vi "valuation.vi"(0 "Input pixmap":i32[][](array[numeric]), 1 "Ref. N.":i32) -> (2 "4-bit pixmap 3":u8[][](array[numeric])=[[0, 0, 0, 0, 0, 0, 0, 0, 0, 0, 0, 0, 0, 0, 0, 0, 0, 0, 0, 0, 0, 0, 0], [0, 0, 0, 0, 0, 1, 1, 1, 1, 1, 0, 0, 0, 0, 0, 0, 1, 1, 1, 1, 1, 1, 0], [0, 0, 0, 0, 1, 1, 1, 1, 1, 1, 1, 1, 0, 0, 0, 1, 1, 1, 1, 1, 1, 1, 0], [0, 0, 0, 1, 1, 1, 1, 1, 1, 1, 1, 1, 1, 0, 1, 1, 1, 1, 1, 1, 1, 1, 0], [0, 0, 1, 1, 1, 1, 0, 0, 0, 1, 1, 1, 1, 0, 1, 1, 1, 1, 0, 0, 0, 0, 0], [0, 0, 1, 1, 1, 1, 0, 0, 0, 1, 1, 1, 1, 0, 1, 1, 1, 0, 0, 0, 0, 0, 0], [0, 0, 1, 1, 1, 1, 0, 0, 0, 1, 1, 1, 1, 1, 1, 1, 1, 1, 1, 1, 0, 0, 0], [0, 0, 1, 1, 1, 1, 0, 0, 0, 1, 1, 1, 1, 1, 1, 1, 1, 1, 1, 1, 1, 0, 0], [0, 0, 1, 1, 1, 1, 1, 1, 1, 1, 1, 1, 0, 1, 1, 0, 0, 1, 1, 1, 1, 1, 0], [0, 0, 0, 1, 1, 1, 1, 1, 1, 1, 1, 1, 0, 0, 0, 0, 0, 0, 1, 1, 1, 1, 0], [0, 0, 0, 0, 0, 1, 1, 1, 1, 1, 1, 0, 0, 0, 0, 0, 0, 0, 1, 1, 1, 1, 0], [0, 0, 0, 0, 0, 0, 1, 1, 1, 1, 0, 0, 1, 0, 0, 0, 0, 0, 1, 1, 1, 1, 0], [0, 0, 0, 0, 0, 1, 1, 1, 1, 0, 0, 1, 1, 1, 1, 0, 0, 1, 1, 1, 1, 0, 0], [0, 0, 0, 0, 1, 1, 1, 1, 0, 0, 0, 1, 1, 1, 1, 1, 1, 1, 1, 1, 1, 0, 0], [0, 0, 0, 0, 1, 1, 1, 0, 0, 0, 0, 0, 1, 1, 1, 1, 1, 1, 1, 1, 0, 0, 0], [0, 0, 0, 0, 0, 0, 0, 0, 0, 0, 0, 0, 0, 0, 0, 0, 0, 0, 0, 0, 0, 0, 0], [0, 0, 0, 0, 0, 0, 0, 0, 0, 0, 0, 0, 0, 0, 0, 0, 0, 0, 0, 0, 0, 0, 0], [0, 0, 0, 0, 0, 0, 0, 0, 0, 0, 0, 0, 0, 0, 0, 0, 0, 0, 0, 0, 0, 0, 0], [0, 0, 0, 0, 0, 0, 0, 0, 0, 0, 0, 0, 0, 0, 0, 0, 0, 0, 0, 0, 0, 0, 0]] caption="ref. Number" format="%#.1f", 4 "ref. picture":picture caption="ref. pic.", 5 "matched pixmap":i32[][](array[numeric]), 6 "total identify %":dbl format="%#_3g", 7 "vertical × yoko":i32[](array[numeric]))   [LabVIEW 2016]
uses:
  <vilib>/picture/picture.llb/imagedata.ctl
panel:
  out "image data 2":T1 caption="画像データ"
  in  "value method":bool
  in  "タブ制御器":enum32{"picture", "array", "expand"}(tab)
  out "input picture 2":picture caption="Input pic."
  out "new picture":picture caption="matched pic."
  out "image data":T1 caption="画像データ"
  out "input data":T1 caption="画像データ"
  out "map N":i32
  out "sample blackN":i32
  out "ref. data 2":T1 caption="画像データ"
  out "Ref. blackN":i32
  out "sample     ref.  identify":dbl[](array[numeric]) format="%#_3g"
  out "new picture 2":picture caption="falsepix pic."
  out "Expand test pic. 3":picture caption="naname Expanded pic."
  out "unmatched pixmap":i32[][](array[numeric])
  # "1/0"
  # "updown"
  # "="
  # "white : matched\nyellow : only samp. \nblack : only Ref."
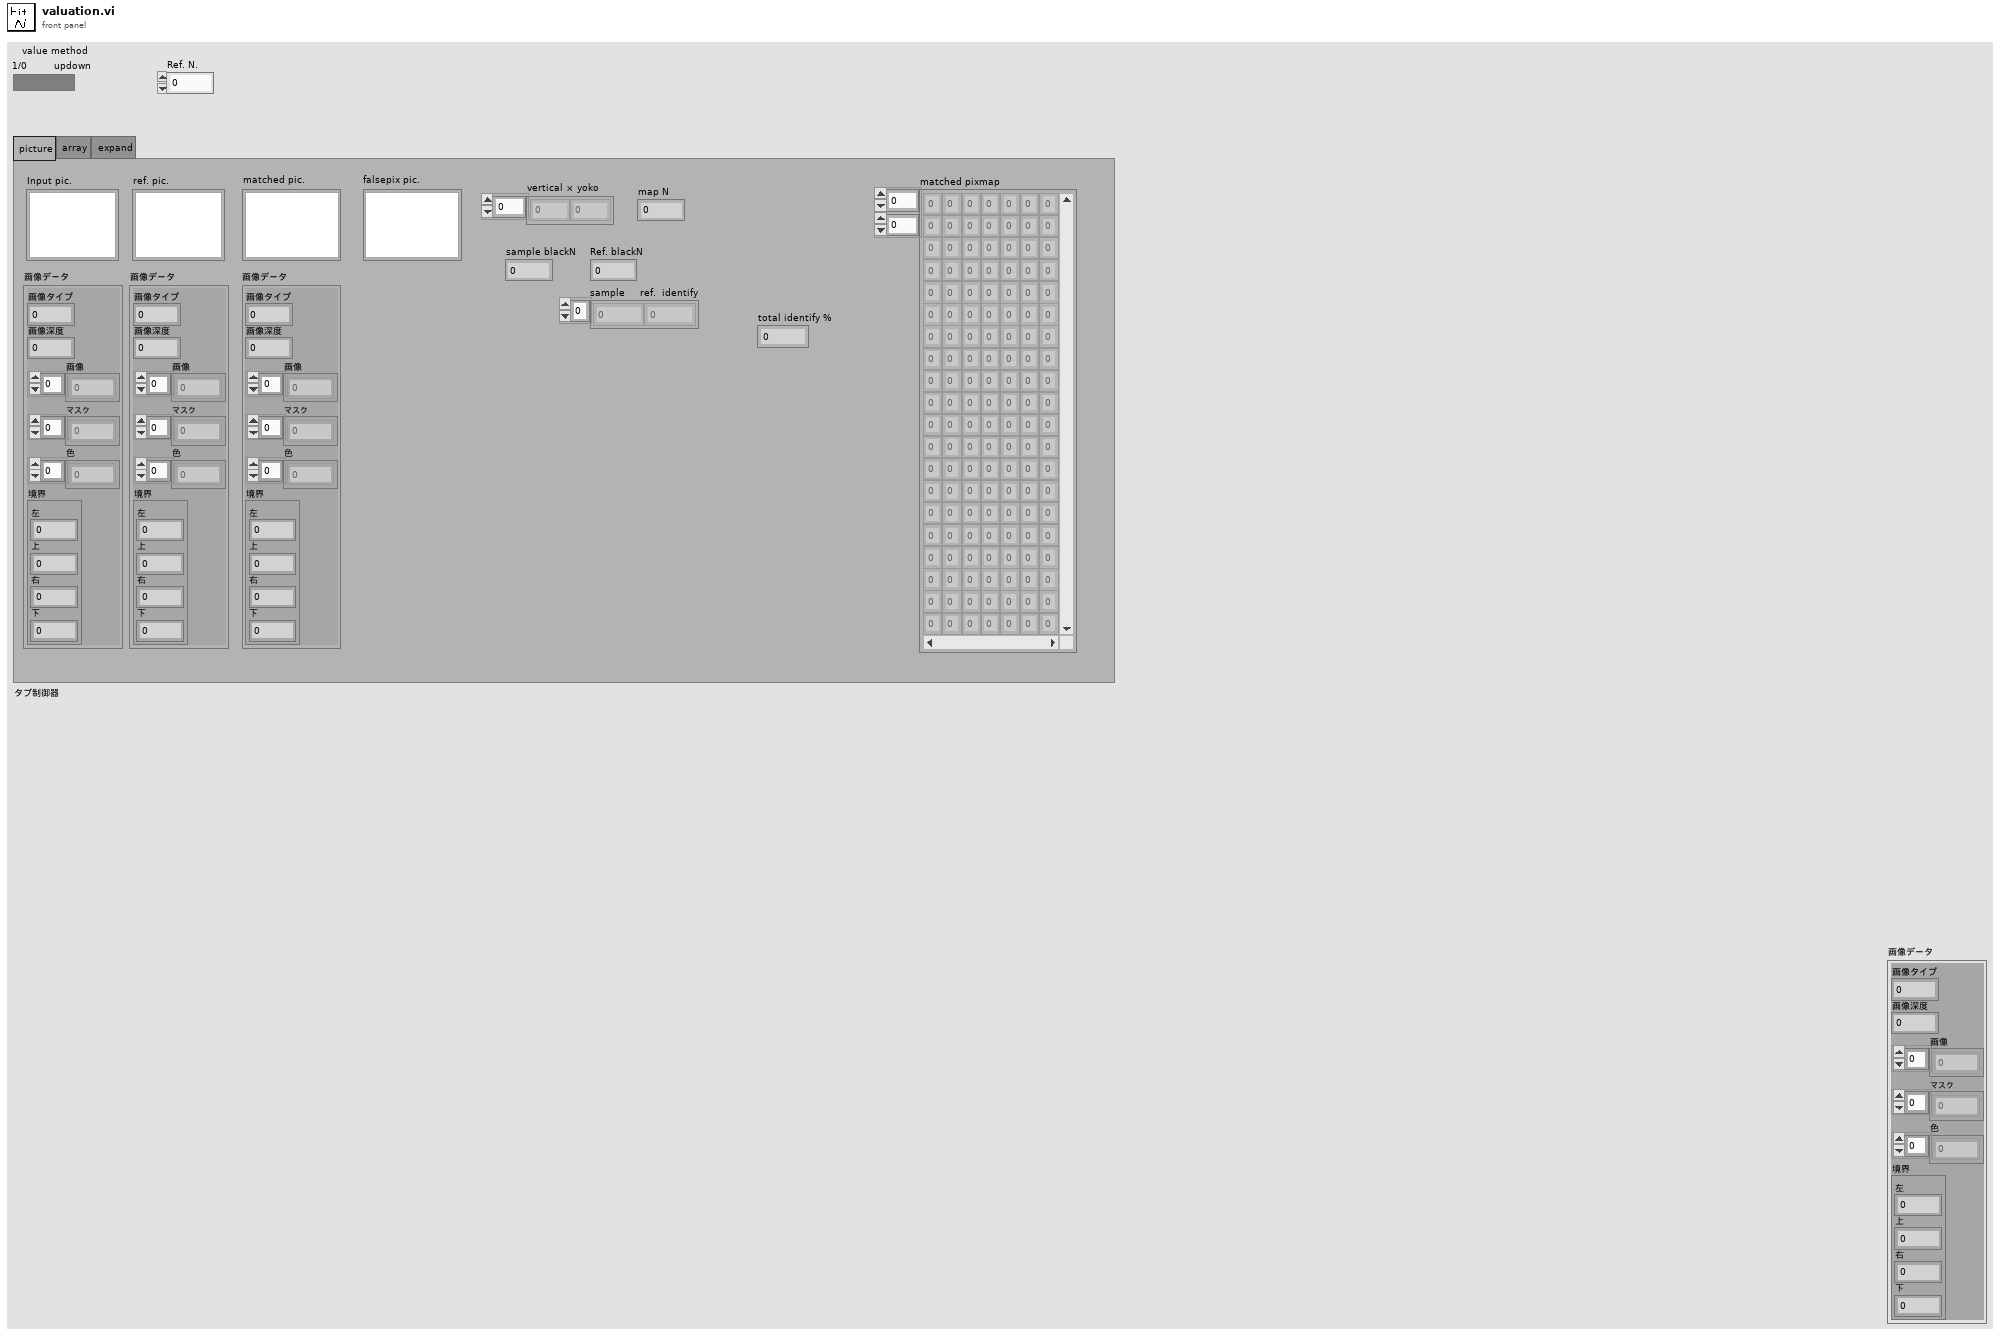
[diagram p1: front panel]
types:
  T1 = typedef "imagedata.ctl" = cluster{"image type":i32, "image depth":i32, "image":u8[], "mask":u8[], "colors":u32[], "Rectangle":cluster{"left":i16, "top":i16, "right":i16, "bottom":i16}}
  T2 = typedef "LVBoundsTypeDef.ctl" = cluster{"Width":u32, "Height":u32}
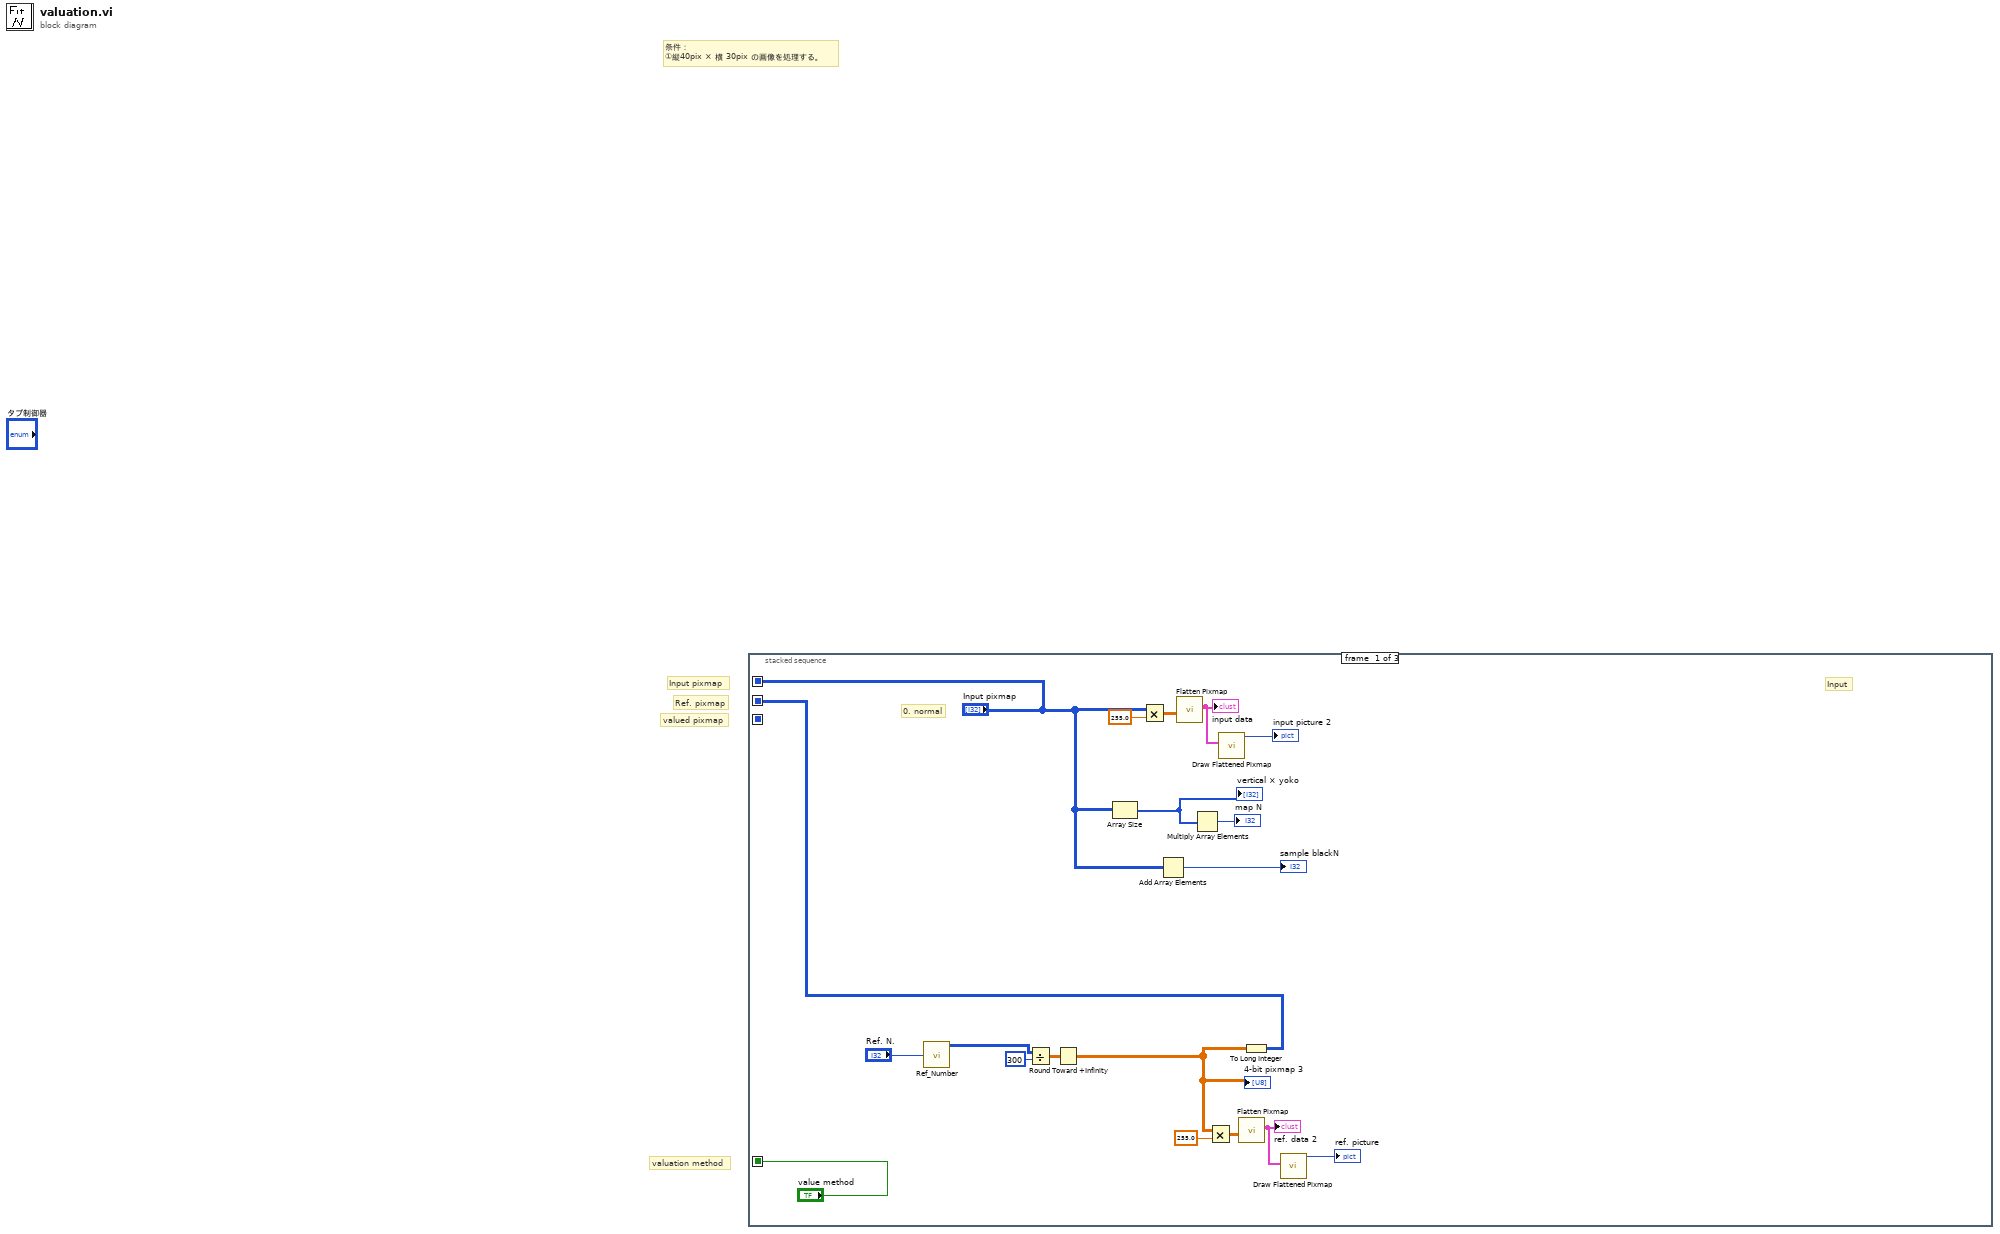
[diagram p0: block diagram]
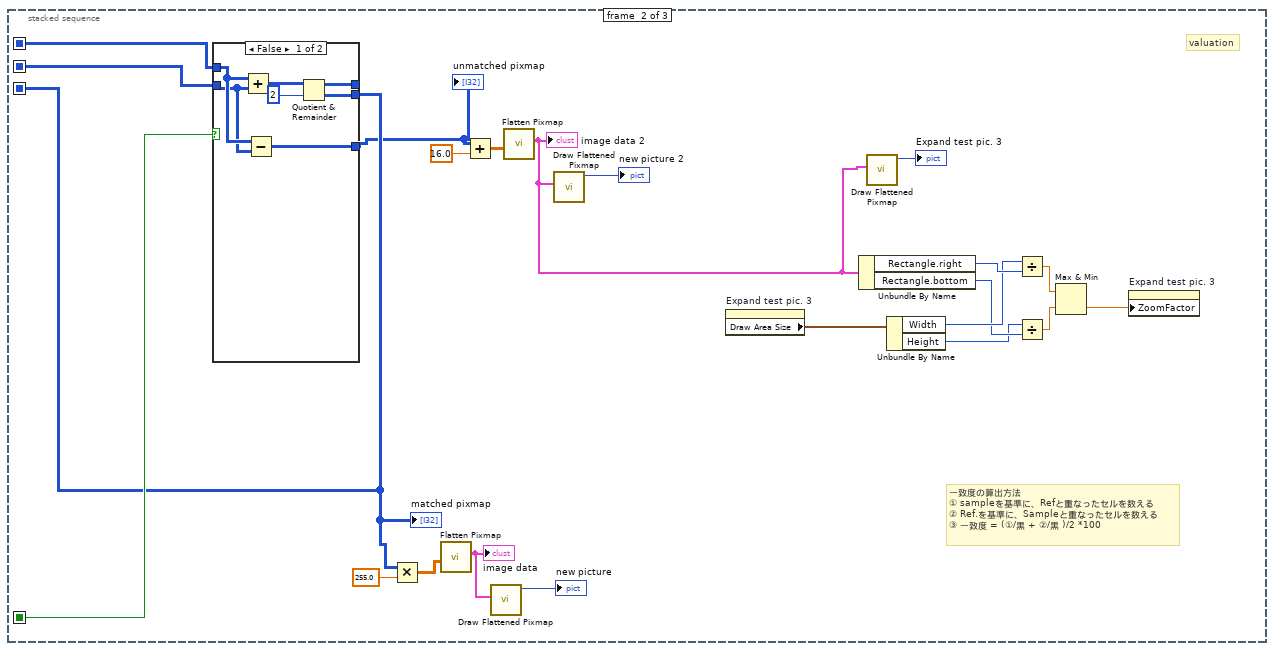
[diagram p2: hidden frame]
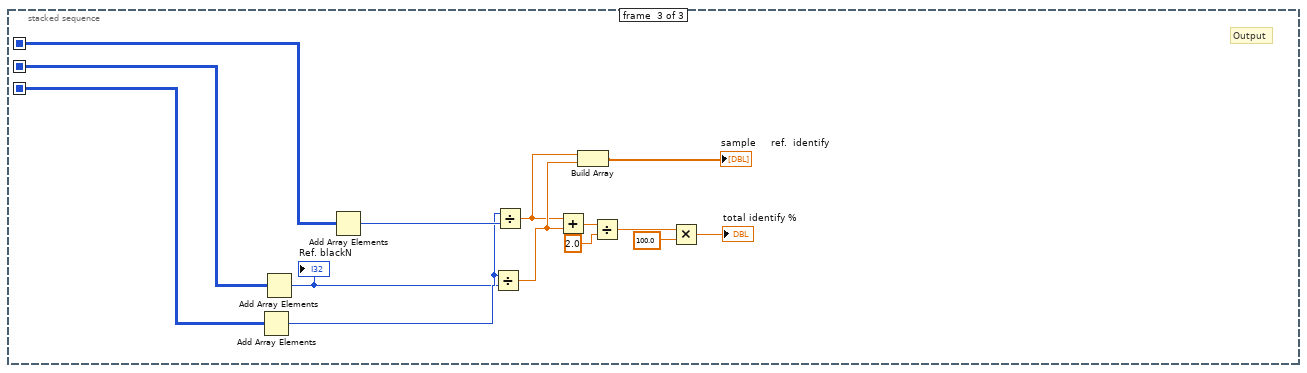
[diagram p4: hidden frame]
diagram:
  # "valued pixmap"
  # "valuation method"
  # "Ref. pixmap"
  # "Input pixmap"
  # "条件：\n①縦40pix × 横 30pix の画像を処理する。"
  n1 = stacked-sequence {
    seq-local: ["Input pixmap" _ _] -> [_ w40 w53]
    seq-local: [w6 _ _] -> [_ w41 w52]
    seq-local: ["value method" _ _] -> [_ w39 _]
    seq-local: [_ w34 _] -> [_ _ w51]
    frame #0 {
      # "Input"
      # "0. normal"
      n2 = call "Ref_Number.vi"("inform N."="Ref. N.") -> ("Output bitmap"=w4:u8[][])  [unwired: 3 out]
      n3 = Divide(x=w4, y=300) -> (x/y=w2:dbl[][])
      n4 = Round Toward +Infinity(x=w2) -> (ceil(x): smallest int >= x=w1:dbl[][])
      "4-bit pixmap 3" <- w1
      n5 = Array Size(array="Input pixmap") -> (size(s)=w8:i32[])
      "vertical × yoko" <- w8
      n6 = Multiply(x="Input pixmap", y=255.0) -> (x*y=w14:dbl[][])
      n7 = Add Array Elements(numeric array="Input pixmap") -> (sum=→"sample blackN":i32)
      n8 = call <vilib>:"Flatten Pixmap.vi"("4-bit pixmap"=w14) -> ("image data"=w11:T1)  [unwired: 10 in]
      "input data" <- w11
      n9 = Multiply Array Elements(1:w8) -> (0:→"map N":i32)
      n10 = Multiply(x=w1, y=255.0) -> (x*y=w18:dbl[][])
      n11 = call <vilib>:"Draw Flattened Pixmap.vi"("image data"=w11) -> ("new picture"=→"input picture 2":picture)  [unwired: 8 in]
      n12 = call <vilib>:"Flatten Pixmap.vi"("4-bit pixmap"=w18) -> ("image data"=w15:T1)  [unwired: 10 in]
      "ref. data 2" <- w15
      n13 = To Long Integer(number=w1) -> (32bit integer=w6:i32[][])
      n14 = call <vilib>:"Draw Flattened Pixmap.vi"("image data"=w15) -> ("new picture"=→"ref. picture":picture)  [unwired: 8 in]
    }
    frame #1 {
      # "valuation"
      # "一致度の算出方法\n① sampleを基準に、Refと重なったセルを数える\n② Ref.を基準に、Sampleと重なったセルを数える\n③ 一致度 = (①/黒 + ②/黒 )/2 *100"
      n15 = case shown="False" w39 {
        tunnel: [w48 _] -> w34
        tunnel: w41 -> [w43 _]
        tunnel: w40 -> [w44 _]
        tunnel: [w45 _] -> _
        tunnel: [w42 _] -> w30
        frame False {
          n16 = Add(x=w44, y=w43) -> (x+y=w46:i32[][])
          n17 = Subtract(x=w44, y=w43) -> (x-y=w42:i32[][])
          n18 = Quotient & Remainder(x=w46, y=2) -> (x-y*floor(x/y)=w45:i32[][], floor(x/y)=w48:i32[][])
        }
        frame True {
        }
      }
      "matched pixmap" <- w34
      "unmatched pixmap" <- w30
      n19 = Multiply(x=w34, y=255.0) -> (x*y=w38:dbl[][])
      n20 = call <vilib>:"Flatten Pixmap.vi"("4-bit pixmap"=w38) -> ("image data"=w35:T1)  [unwired: 10 in]
      "image data" <- w35
      n21 = Add(x=w30, y=16.0) -> (x+y=w32:dbl[][])
      n22 = call <vilib>:"Draw Flattened Pixmap.vi"("image data"=w35) -> ("new picture"=→"new picture":picture)  [unwired: 8 in]
      n23 = call <vilib>:"Flatten Pixmap.vi"("4-bit pixmap"=w32) -> ("image data"=w20:T1)  [unwired: 10 in]
      "image data 2" <- w20
      n24 = call <vilib>:"Draw Flattened Pixmap.vi"("image data"=w20) -> ("new picture"=→"new picture 2":picture)  [unwired: 8 in]
      n25 = property on="Expand test pic. 3" class="Pict"() -> ("Draw Area Size"=w29:T2)  [unwired: 2 in, 2 out]
      n26 = Unbundle By Name(w20) -> ("Rectangle.right"=w28:i16, "Rectangle.bottom"=w26:i16)
      n27 = call <vilib>:"Draw Flattened Pixmap.vi"("image data"=w20) -> ("new picture"=→"Expand test pic. 3":picture)  [unwired: 8 in]
      n28 = Unbundle By Name(w29) -> ("Width"=w27:u32, "Height"=w25:u32)
      n29 = Divide(x=w27, y=w28) -> (x/y=w23:dbl)
      n30 = Divide(x=w25, y=w26) -> (x/y=w24:dbl)
      n31 = Max & Min(x=w23, y=w24) -> (min(x,y)=w22:dbl)  [unwired: 1 out]
      n32 = property on="Expand test pic. 3" class="Pict"("ZoomFactor"=w22) -> ()  [unwired: 2 in, 2 out]
    }
    frame #2 {
      # "Output"
      n33 = Add Array Elements(numeric array=w51) -> (sum=w50:i32)
      n34 = Add Array Elements(numeric array=w52) -> (sum=w49:i32)
      "Ref. blackN" <- w49
      n35 = Add Array Elements(numeric array=w53) -> (sum=w54:i32)
      n36 = Divide(x=w50, y=w49) -> (x/y=w60:dbl)
      n37 = Divide(x=w50, y=w54) -> (x/y=w59:dbl)
      n38 = Add(x=w59, y=w60) -> (x+y=w56:dbl)
      n39 = Build Array(w59, w60) -> (→"sample     ref.  identify":dbl[])
      n40 = Divide(x=w56, y=2.0) -> (x/y=w58:dbl)
      n41 = Multiply(x=w58, y=100.0) -> (x*y=→"total identify %":dbl)
    }
  }
